vi "2D_Session_Data.vi"(9 "Iteration":i32, 10 "Session":i32) -> (2 "output cluster":T1)   [LabVIEW 2011]
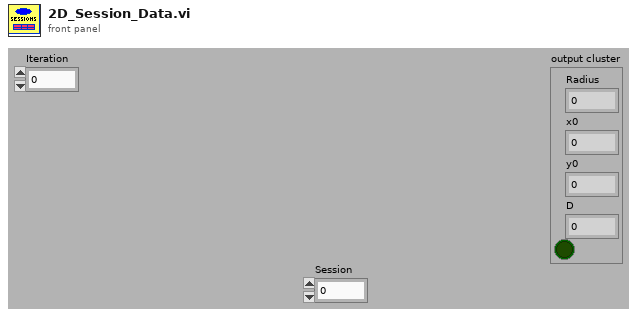
[diagram p1: front panel]
types:
  T1 = cluster{"Radius":dbl, "x0":dbl, "y0":dbl, "D":dbl, bool}
  T2 = cluster{"Radius":dbl, "x0":dbl, "x0":dbl, "x0":dbl, bool}
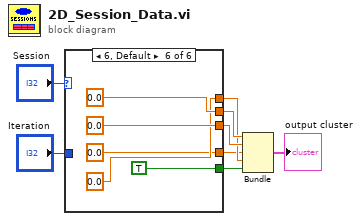
[diagram p0: block diagram]
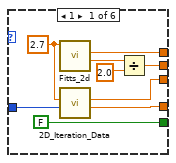
[diagram p2: hidden frame]
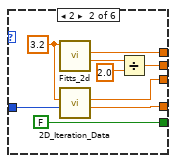
[diagram p3: hidden frame]
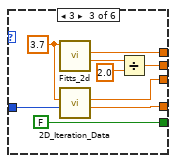
[diagram p4: hidden frame]
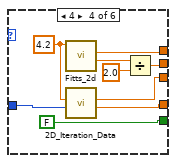
[diagram p5: hidden frame]
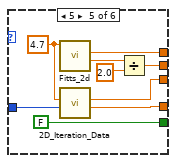
[diagram p6: hidden frame]
diagram:
  n1 = case shown="6, Default" "Session" {
    tunnel: [w16 w23 w32 w39 w50 0.0 ("Radius")] -> w7
    tunnel: [w10 w20 w30 w38 w48 0.0 ("x0")] -> w6
    tunnel: [w13 w18 w28 w40 w46 0.0 ("x0")] -> w5
    tunnel: [FALSE FALSE FALSE FALSE FALSE TRUE] -> w4
    tunnel: [w9 w19 w29 w37 w47 0.0 ("x0")] -> w3
    tunnel: "Iteration" -> [w12 w22 w31 w41 w49 _]
    frame 1 {
      w11 = 2.7 ("ID")
      n2 = call "Fitts_2d.vi"("ID"=w11) -> ("W"=w14:dbl, "D"=w13:dbl)  [unwired: 9 in]
      n3 = call "2D_Iteration_Data.vi"("Iteration"=w12, "ID"=w11) -> ("y0"=w9:dbl, "x0"=w10:dbl)  [unwired: 8 in]
      n4 = Divide(x=w14, y=2.0) -> (x/y=w16:dbl)
    }
    frame 2 {
      w21 = 3.2 ("ID")
      n5 = call "Fitts_2d.vi"("ID"=w21) -> ("W"=w24:dbl, "D"=w18:dbl)  [unwired: 9 in]
      n6 = call "2D_Iteration_Data.vi"("Iteration"=w22, "ID"=w21) -> ("y0"=w19:dbl, "x0"=w20:dbl)  [unwired: 8 in]
      n7 = Divide(x=w24, y=2.0) -> (x/y=w23:dbl)
    }
    frame 3 {
      w27 = 3.7 ("ID")
      n8 = call "Fitts_2d.vi"("ID"=w27) -> ("W"=w33:dbl, "D"=w28:dbl)  [unwired: 9 in]
      n9 = call "2D_Iteration_Data.vi"("Iteration"=w31, "ID"=w27) -> ("y0"=w29:dbl, "x0"=w30:dbl)  [unwired: 8 in]
      n10 = Divide(x=w33, y=2.0) -> (x/y=w32:dbl)
    }
    frame 4 {
      w42 = 4.2 ("ID")
      n11 = call "Fitts_2d.vi"("ID"=w42) -> ("W"=w43:dbl, "D"=w40:dbl)  [unwired: 9 in]
      n12 = call "2D_Iteration_Data.vi"("Iteration"=w41, "ID"=w42) -> ("y0"=w37:dbl, "x0"=w38:dbl)  [unwired: 8 in]
      n13 = Divide(x=w43, y=2.0) -> (x/y=w39:dbl)
    }
    frame 5 {
      w45 = 4.7 ("ID")
      n14 = call "Fitts_2d.vi"("ID"=w45) -> ("W"=w51:dbl, "D"=w46:dbl)  [unwired: 9 in]
      n15 = call "2D_Iteration_Data.vi"("Iteration"=w49, "ID"=w45) -> ("y0"=w47:dbl, "x0"=w48:dbl)  [unwired: 8 in]
      n16 = Divide(x=w51, y=2.0) -> (x/y=w50:dbl)
    }
    frame 6, Default {
    }
  }
  n17 = Bundle("Radius"=w7, "x0"=w6, "x0"=w3, "x0"=w5, w4) -> (→"output cluster":T2)  [unwired: 1 in]
